vi "GetDisplayUsableBounds.vi"(8 "No Error":errorcluster, 11 "Display ID":T2) -> (0 "Error Out":errorcluster, 3 "Display Usable Bounds":T1)   [LabVIEW 2026, in "SDL3.lvlib" / "Video.lvlib"]
doc: "<B>Summary</B>\nGet the usable desktop area represented by a display, in screen coordinates.\n\n<B>Remarks</B>\nThis is the same area as SDL_GetDisplayBounds() reports, but with portions reserved by the system removed. For example, on Apple's macOS, this subtracts the area occupied by the menu bar and dock.\n\nSetting a window to be fullscreen generally bypasses these unusable areas, so these are good guidelines for the maximum space available to a non-fullscreen window."
uses:
  Video.lvlib
  DisplayID--integer.ctl
  Rect/Rect--cluster.ctl
  <vilib>/Utility/error.llb/Error Cluster From Error Code.vi
  Rect/Rect.lvlib
  Error/Error.lvlib
  Lib/SDL3.dll
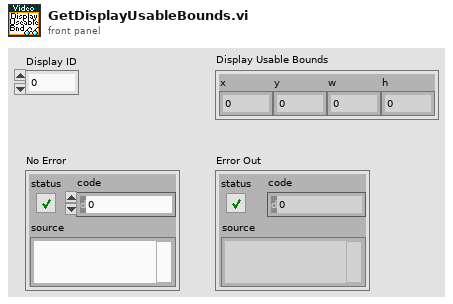
[diagram p1: front panel]
types:
  T1 = typedef "SDL3.lvlib/Rect.lvlib/Rect--cluster.ctl" = cluster{"x":i32, "y":i32, "w":i32, "h":i32}
  T2 = typedef "SDL3.lvlib/Video.lvlib/DisplayID--integer.ctl" = u32
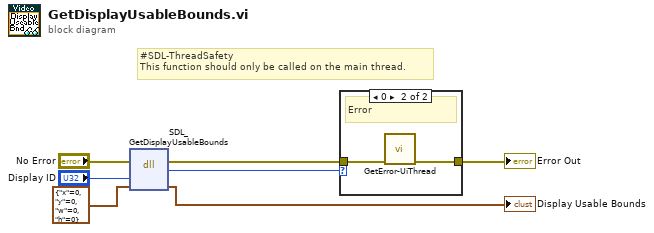
[diagram p0: block diagram]
diagram:
  # "#SDL-ThreadSafety\nThis function should only be called on the main thread."
  n1 = dll-call lib="C:/Users/saukko/Dev/LV-SDL3/Sources/SDL3/Lib/SDL3.*" fn="SDL_GetDisplayUsableBounds"(error in="No Error", "displayID"="Display ID", "rect"=T1 {"x"=0, "y"=0, "w"=0, "h"=0} ("Display Usable Bounds")) -> (error out=w5:errorcluster, "return type"=w1:i32, "rect"=→"Display Usable Bounds":T1)  [unwired: 3 in, 1 out]
  n2 = case shown="0" w1 {
    tunnel: w5 -> [w8 w10]
    tunnel: [w8 w9] -> w6
    frame Default {
      # "Ok"
    }
    frame 0 {
      # "Error"
      n3 = call "GetError-UiThread.vi"("No Error"=w10) -> ("error out"=w9:errorcluster)  [unwired: 10 in]
    }
  }
  "Error Out" <- w6
